vi "Configure Protect Clear.vi"(8 "error in (no error)":errorcluster, 11 "VISA resource name":refnum<visa-resource-name>) -> (0 "error out":errorcluster, 3 "VISA resource name out":refnum<visa-resource-name>)   [LabVIEW 2020, in "IT6500.lvlib"]
doc: "This command is used to remove overvoltage protection.After this command is executed, the output voltage will be restored\nOVP protection occurs before the output state and the upper voltage value of the OVP overvoltage protection remains unchanged\nSet the value.Before sending this command, the output voltage is reduced to below the OVP upper voltage value,\nOr increase the upper voltage value of the OVP.Also notice that the external power source that causes overvoltage protection should be removed first\nSend this command again."
uses:
  IT6500.lvlib
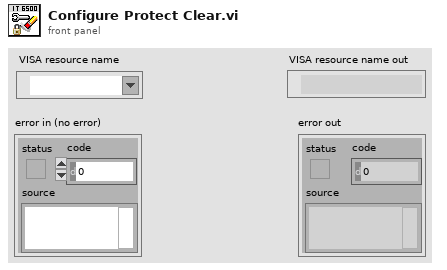
[diagram p1: front panel]
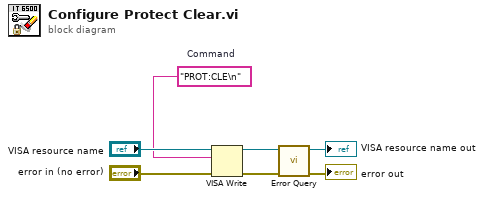
[diagram p0: block diagram]
diagram:
  w5 = "PROT:CLE\n"  # Command
  n1 = VISA Write(VISA resource name="VISA resource name", write buffer=w5, error in (no error)="error in (no error)") -> (VISA resource name out=w3:refnum<visa-resource-name>, error out=w4:errorcluster)  [unwired: 1 out]
  n2 = call "Error Query.vi"("error in (no error)"=w4, "VISA resource name"=w3) -> ("error out"=→"error out":errorcluster, "VISA resource name out"=→"VISA resource name out":refnum<visa-resource-name>)  [unwired: 6 in, 2 out]
